vi "create_pack.vi"(2 "error in":errorcluster) -> (0 "error out":errorcluster, 1 "p":u64)   [LabVIEW 2019, in "msgpack.lvlib"]
doc: "Allocates memory for a msgpack packing object, returned in the pointer p"
uses:
  msgpack.lvlib
  msgpackalt.dll
panel:
  # "msgpack"
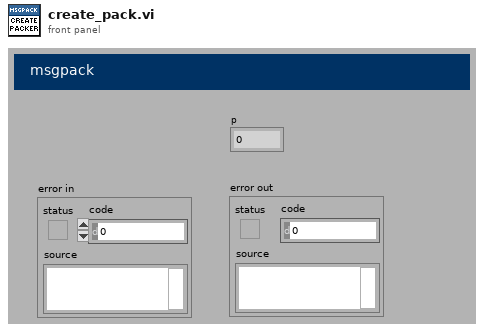
[diagram p1: front panel]
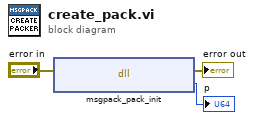
[diagram p0: block diagram]
diagram:
  n1 = dll-call lib="C:/Users/Patrick/Documents/GitHub/Instrument-Framework/lvsrc/SMOs/JSON-RPC-2019/lv-venv/lv.lib/vi.lib/addons/msgpack/msgpackalt.dll" fn="msgpack_pack_init"(error in="error in") -> (error out=→"error out":errorcluster, "return type"=→"p":u64)  [unwired: 2 in, 1 out]
